vi "MainE.vi"   [LabVIEW 2023, in "ModuleE.lvlib"]
uses:
  ModuleE.lvlib
  ModuleF.lvlib
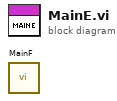
[diagram p0: block diagram]
diagram:
  n1 = call "MainF.vi"() -> ()  [unwired: 12 in]
